vi "endEventToStringArray.vi"(8 "error in (no error)":errorcluster, 11 "RampUp in":refnum<class "RampUp.lvclass">) -> (0 "error out":errorcluster, 2 "eventStringArray":string[](array[string]), 3 "RampUp out":refnum<class "RampUp.lvclass">)   [LabVIEW 2009, in "Tools.lvlib" / "Scripting.lvlib" / "RampUp.lvclass"]
uses:
  RampUp.lvclass
  ScriptEvent.lvclass
  RampEvent/RampEvent.lvclass
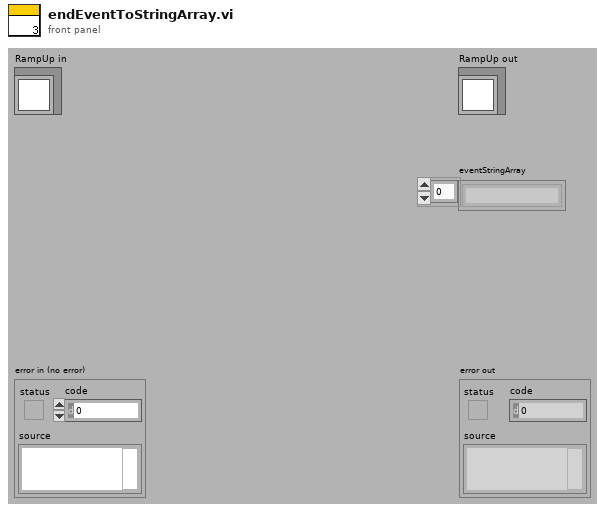
[diagram p1: front panel]
types:
  T1 = cluster{"rampTime":dbl, "timeStep":dbl, "dataValueStep":dbl}
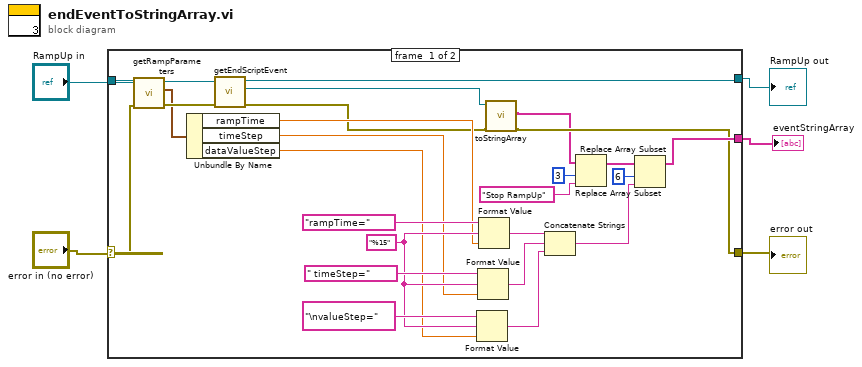
[diagram p0: block diagram]
diagram:
  n1 = case shown="No Error" "error in (no error)" {
    selector: "error in (no error)" -> [w6 w32]
    tunnel: [w11 w33] -> w3
    tunnel: "RampUp in" -> [w15 w33]
    tunnel: [w10 w32] -> w1
    tunnel: [w16 _] -> w2
    frame #0 {
      w28 = "%15"
      n2 = call "getRampParameters.vi"("error in (no error)"=w6, "RampEvent in"=w15) -> ("error out"=w13:errorcluster, "RampParameters"=w12:T1, "RampEvent out"=w14:refnum<class "RampUp.lvclass">)  [unwired: 7 in]
      n3 = Unbundle By Name(w12) -> ("rampTime"=w19:dbl, "timeStep"=w18:dbl, "dataValueStep"=w17:dbl)
      n4 = call "getEndScriptEvent.vi"("error in (no error)"=w13, "RampEvent.lvclass in"=w14) -> ("error out"=w7:errorcluster, "ScriptEvent.lvclass"=w9:refnum<class "ScriptEvent.lvclass">, "RampEvent.lvclass out"=w11:refnum<class "RampUp.lvclass">)  [unwired: 7 in]
      n5 = Format Value(string ("")="\nvalueStep=", format string=w28, value (0)=w17) -> (output string=w21:string)
      n6 = Format Value(string ("")=" timeStep=", format string=w28, value (0)=w18) -> (output string=w22:string)
      n7 = Format Value(string ("")="rampTime=", format string=w28, value (0)=w19) -> (output string=w23:string)
      n8 = call-dynamic "toStringArray.vi"("error in (no error)"=w7, "ScriptEvent in"=w9) -> ("error out"=w10:errorcluster, "eventStringArray"=w8:string[])  [unwired: 7 in, 1 out]
      n9 = Concatenate Strings(w23, w22, w21) -> (w20:string)
      n10 = Replace Array Subset(array=w8, new element="Stop RampUp", index=3) -> (w26:string[])
      n11 = Replace Array Subset(array=w26, new element=w20, index=6) -> (w16:string[])
    }
    frame #1 {
    }
  }
  "error out" <- w1
  "RampUp out" <- w3
  "eventStringArray" <- w2
